vi "Engine-CreateWindow.vi"(8 "error in (no error)":errorcluster, 11 "Window in":refnum<class "Window.lvclass">) -> (0 "error out":errorcluster, 1 "Window ID":T1, 2 "Window [SDL_Window *]":i64, 3 "Window out":refnum<class "Window.lvclass">)   [LabVIEW 2020, in "GLF.lvlib" / "Window.lvclass"]
uses:
  Window.lvclass
  Window.lvclass/Window.ctl
  <vilib>/Saukko/LV SDL3/Sources/SDL3/Video/Video.lvlib
  <vilib>/Saukko/LV SDL3/Sources/SDL3/Video/WindowFlags--ring.ctl
  <vilib>/Saukko/LV SDL3/Sources/SDL3/Video/WindowID--integer.ctl
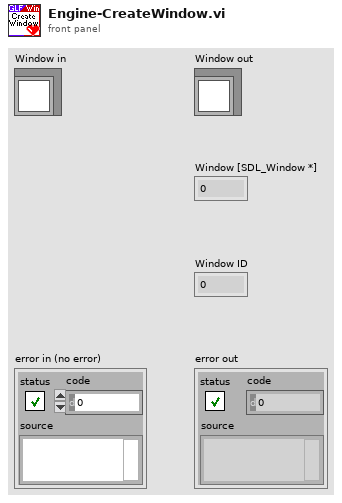
[diagram p1: front panel]
types:
  T1 = typedef "SDL3.lvlib/Video.lvlib/WindowID--integer.ctl" = u32
  T2 = typedef "SDL3.lvlib/Video.lvlib/WindowFlags--ring.ctl" = u64
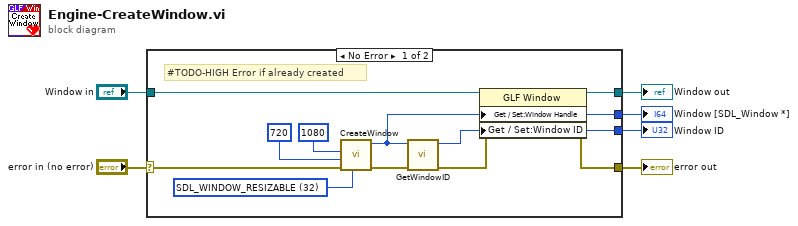
[diagram p0: block diagram]
diagram:
  n1 = case shown="No Error" "error in (no error)" {
    selector: "error in (no error)" -> [w16 w19]
    tunnel: [w17 w19] -> w5
    tunnel: [w11 w18] -> w3
    tunnel: "Window in" -> [w12 w18]
    tunnel: [w8 _] -> w2
    tunnel: [w7 _] -> w1
    frame No Error {
      w13 = T2 32 items=["0"=0, "SDL_WINDOW_FULLSCREEN"=1, "SDL_WINDOW_OPENGL"=2, "SDL_WINDOW_OCCLUDED"=4, "SDL_WINDOW_HIDDEN"=8, "SDL_WINDOW_BORDERLESS"=16, "SDL_WINDOW_RESIZABLE"=32, "SDL_WINDOW_MINIMIZED"=64, "SDL_WINDOW_MAXIMIZED"=128, "SDL_WINDOW_MOUSE_GRABBED"=256, "SDL_WINDOW_INPUT_FOCUS"=512, "SDL_WINDOW_MOUSE_FOCUS"=1024, "SDL_WINDOW_EXTERNAL"=2048, "SDL_WINDOW_MODAL"=4096, "SDL_WINDOW_HIGH_PIXEL_DENSITY"=8192, "SDL_WINDOW_MOUSE_CAPTURE"=16384, "SDL_WINDOW_MOUSE_RELATIVE_MODE"=32768, "SDL_WINDOW_ALWAYS_ON_TOP"=65536, "SDL_WINDOW_UTILITY"=131072, "SDL_WINDOW_TOOLTIP"=262144, "SDL_WINDOW_POPUP_MENU"=524288, "SDL_WINDOW_KEYBOARD_GRABBED"=1048576, "SDL_WINDOW_VULKAN"=268435456, "SDL_WINDOW_METAL"=536870912, "SDL_WINDOW_TRANSPARENT"=1073741824, "SDL_WINDOW_NOT_FOCUSABLE"=2147483648] ("flags (0)")
      # "#TODO-HIGH Error if already created"
      n2 = call <vilib>:"CreateWindow.vi"("Flags (0)"=w13, "No Error"=w16, "h"=720, "w"=1080) -> ("Error Out"=w10:errorcluster, "Window [SDL_Window *]"=w8:i64)  [unwired: 6 in]
      n3 = call <vilib>:"GetWindowID.vi"("No Error"=w10, "Window [SDL_Window *]"=w8) -> ("Error Out"=w9:errorcluster, "Window ID"=w7:T1)  [unwired: 8 in]
      n4 = property class="GLF Window"(reference=w12, error in=w9, "Get / Set:Window Handle"=w8, "Get / Set:Window ID"=w7) -> (reference out=w11:refnum<class "Window.lvclass">, error out=w17:errorcluster)
    }
    frame Error {
    }
  }
  "error out" <- w5
  "Window out" <- w3
  "Window [SDL_Window *]" <- w2
  "Window ID" <- w1
